vi "Get Scalar Configuration.vi"(8 "error in (no error)":errorcluster, 9 "index":i32, 11 "Core Channel Configuration in":refnum<class "Core Channels Configuration.lvclass">) -> (0 "error out":errorcluster, 2 "channel configuration":T1={"name"="Channel", "units"="V", "engine data type"=enum."DBL", "string data type"=enum."DBL", "string offset"=0} {"string offset" format="%d bytes"}, 3 "Core Channel Configuration out":refnum<class "Core Channels Configuration.lvclass">)   [LabVIEW 2017, in "DSF Core.lvlib" / "Core Channels Configuration.lvclass"]
uses:
  Core Channels Configuration.lvclass
  Configuration.ctl
  Typedefs/DSF Data Type.ctl
  Core Channels Configuration.lvclass/Core Channels Configuration.ctl
  DSF Core.lvlib
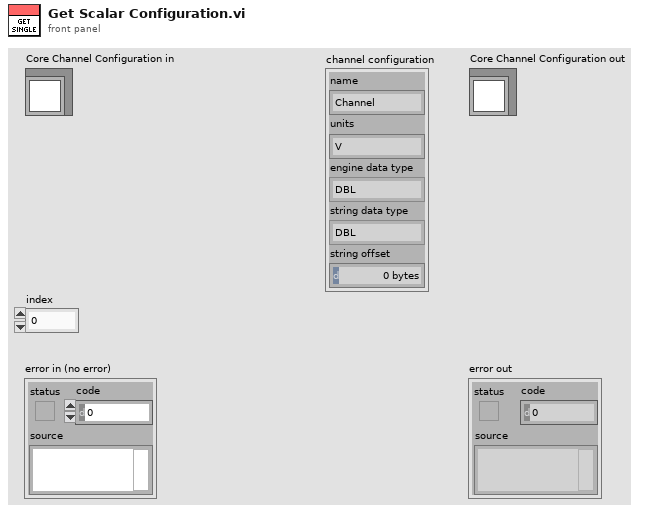
[diagram p1: front panel]
types:
  T1 = typedef "DSF Core.lvlib/Core Channels Configuration.lvclass/Configuration.ctl" = cluster{"name":string, "units":string, "engine data type":T2, "string data type":T2, "string offset":u64}
  T2 = typedef "DSF Core.lvlib/DSF Data Type.ctl" = enum8{"Bool", "SGL", "DBL", "I8", "I16", "I32", "I64", "U8", "U16", "U32", "U64"}
  T3 = typedef "DSF Core.lvlib/Core Channel Configuration.lvclass/Configuration.ctl" = cluster{"name":string, "units":string, "engine data type":T2, "string data type":T2, "string offset":u64}
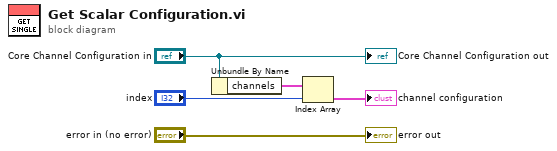
[diagram p0: block diagram]
diagram:
  n1 = Unbundle By Name("Core Channel Configuration in") -> ("channels"=w3:T3[])
  n2 = Index Array(array=w3, index="index") -> (element=→"channel configuration":T3)
  "error out" <- "error in (no error)"
  "Core Channel Configuration out" <- "Core Channel Configuration in"
